vi "FRC Color Processing Example.vi"() -> ()   [LabVIEW 2025]
uses:
  <vilib>/Rock Robotics/WPI/Camera/WPI_CameraSettings Read MJPG.ctl
  <vilib>/Rock Robotics/WPI/Camera/WPI_CameraImageSize.ctl
  Vision Support Code/Camera Types.ctl
  <vilib>/Rock Robotics/WPI/Camera/WPI_CameraExposure Values.ctl
  <vilib>/Rock Robotics/WPI/Camera/WPI_CameraWhite Balance Values.ctl
  <vilib>/vision/NI_Vision_Development_Module.lvlib
panel:
  in  "Line Border":cluster{"Top":dbl, "Bottom":dbl}={"Top"=6.0, "Bottom"=1.0}
  in  "Use Calibration":bool=TRUE
  out "Instructions:":string="Use Source to load image files from a directory, or use a USB or IP camera connected to your laptop. Use Camera Settings 1 and 2 to achieve a dark image with bright and colorful stripes.\nLED Color can encoded as HSL or related color modes. Calibrate to the same color as the strips being reflected to the camera.\nClick and draw a line in Original Image to auto-calibrate the LED Color. You may want to widen and tweak Sat and Val by hand.\nThe Annotate button affects drawing a rectangle around the stripes and labeling it with a distance in ft. Distance relies on knowing the Camera Type and lens calibration (it looks up the lens view angle).\n\nAdjust Score Cutoff to make the code more or less picky. If the color is not very unique, you may need to increase the number of particles considered. The diagram uses a Size Limit to ignore colored things that are too small. You may need to adjust it if you are targetting from far away.\n\nResults give you the distance to the target, the center and box in a normalized (-1 to 1) and pixel coordinates.\n\nBe sure to read about setting camera exposure and brightness to help simplify your image and acquire color saturated images.\n\nThere are lots of comments on the diagram to explain the code."
  in  "Color Mode":u16(ring)=3 items=["RGB", "HSL", "HSV", "HSI"]
  in  "Particles":dbl=5.0
  in  "Score Cutoff %":dbl=70.0
  in  "Std Devs for Calibration":cluster{"H":dbl, "S":dbl, "V":dbl}={"H"=4.0, "S"=6.0, "V"=6.0}
  in  "Camera Type":T1=enum."MS HD3000 square"
  in  "image files":string[](array[string])
  out "Results":T2 {"Score" format="%#_3g"; "Pixels"."Rectangle"."Numeric 5" format="%#_3g"; "Pixels"."Rectangle"."Numeric 3" format="%#_3g"; "Pixels"."Rectangle"."Numeric 2" format="%#_3g"; "Pixels"."Rectangle"."Numeric" format="%#_3g"; "Normalized"."Rectangle"."Numeric 5" format="%#_2g"; "Normalized"."Rectangle"."Numeric 3" format="%#_2g"; "Normalized"."Rectangle"."Numeric 2" format="%#_2g"; "Normalized"."Rectangle"."Numeric" format="%#_2g"; "Normalized"."Center"."?" format="%#_3g"; "Normalized"."Center"."?" format="%#_3g"; "Distance (ft)" format="%#_3g"}
  in  "Source":enum32{"Files", "Camera"}(tab)
  in  "Images":i32(listbox)
  in  "Folder Location":path=path "C:/Program Files (x86)/National Instruments/LabVIEW 2016/examples/FRC/roboRIO/Vision/2017 Vision Example/Sample Images/LED Boiler"
  in  "Camera Settings":T3={"fps"=20, "compression"=30, "Image Size"=enum."320x240", "Config Shown"=FALSE}
  in  "Camera Address":string="USB 1"
  in  "Camera Settings 2":T7={"Exposure"=enum."Auto", "Exposure (%)"=50.0, "Brightness"=50, "White Balance"=enum."Auto", "Color Temp (K)"=0.0} {"Brightness" min=0 max=100}
  in  "Annotate":bool=TRUE
  out "Qualified Particles":i32
  in  "LED Color":T8={"Hue"={107.81818389892578, 139.81818389892578}, "Sat"={176.07142857142858, 255.0}, "Val"={40.53571428571429, 255.0}} {"Hue" scale=0.0..255.0 scale format="%#_3g"}
  out "Mask":T9(plugin-control)
  out "Original Image":T9(plugin-control)
  # "Legend:\n    Rectangle\n       Green - Good target, distance ft\n       Red - Bad target\n    Orange Text - Score in %"
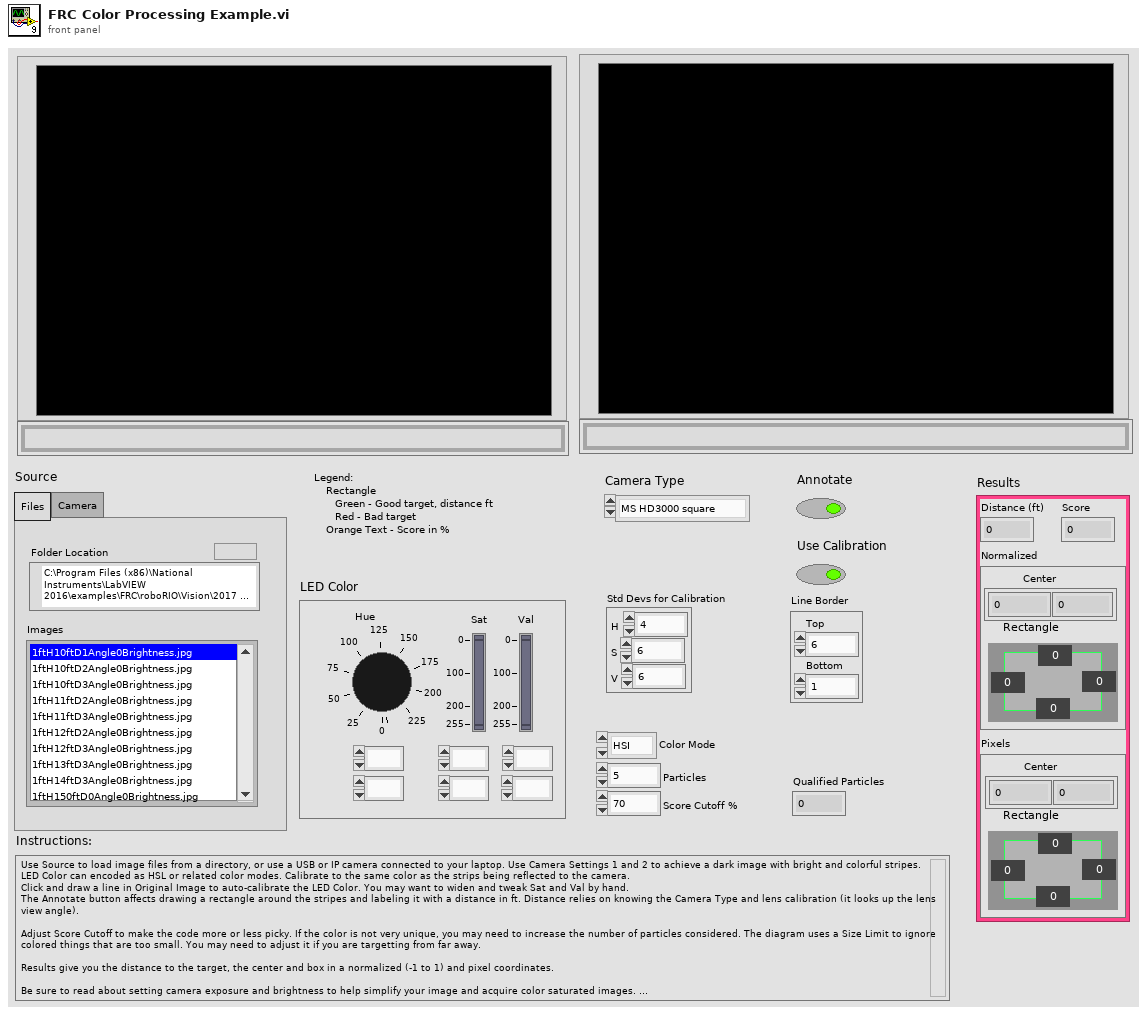
[diagram p1: front panel]
types:
  T1 = typedef "Camera Types.ctl" = enum16{"206", "1011", "1013", "MS HD3000 square", "MS HD3000 640x480"}
  T2 = cluster{"Distance (ft)":dbl, "Score":dbl, "Normalized":cluster{"Center":cluster{dbl, dbl}, "Rectangle":cluster{"Numeric":dbl, "Numeric 2":dbl, "Numeric 3":dbl, "Numeric 5":dbl}}, "Pixels":cluster{"Center":cluster{dbl, dbl}, "Rectangle":cluster{"Numeric":dbl, "Numeric 2":dbl, "Numeric 3":dbl, "Numeric 5":dbl}}}
  T3 = typedef "WPI_CameraSettings Read MJPG.ctl" = cluster{"fps":i32, "compression":i32, "Image Size":T4, "Config Shown":bool}
  T4 = typedef "WPI_CameraImageSize.ctl" = enum16{"640x480", "320x240", "160x120", "Custom"}
  T5 = typedef "WPI_CameraExposure Values.ctl" = enum16{"Auto", "Flicker-free 50 Hz", "Flicker-free 60 Hz", "Hold current", "Custom"}
  T6 = typedef "WPI_CameraWhite Balance Values.ctl" = enum16{"Auto", "Fixed indoor", "Fixed outdoor 1", "Fixed outdoor 2", "Fixed fluorescent 1", "Fixed fluorescent 2", "Hold current", "Custom"}
  T7 = cluster{"Exposure":T5, "Exposure (%)":dbl, "Brightness":i32, "White Balance":T6, "Color Temp (K)":dbl}
  T8 = cluster{"Hue":cluster{dbl, dbl}, "Sat":cluster{dbl, dbl}, "Val":cluster{dbl, dbl}}
  T9 = typedef "IMAQ Image.ctl" = refnum<image>
  T10 = typedef "Image Type" = u32
  T11 = typedef "Particle Parameters" = i32
  T12 = cluster{cluster{dbl, dbl}, cluster{dbl, dbl}, cluster{dbl, dbl}}
  T13 = cluster{"Left":dbl, "Top":dbl, "Right":dbl, "Bottom":dbl}
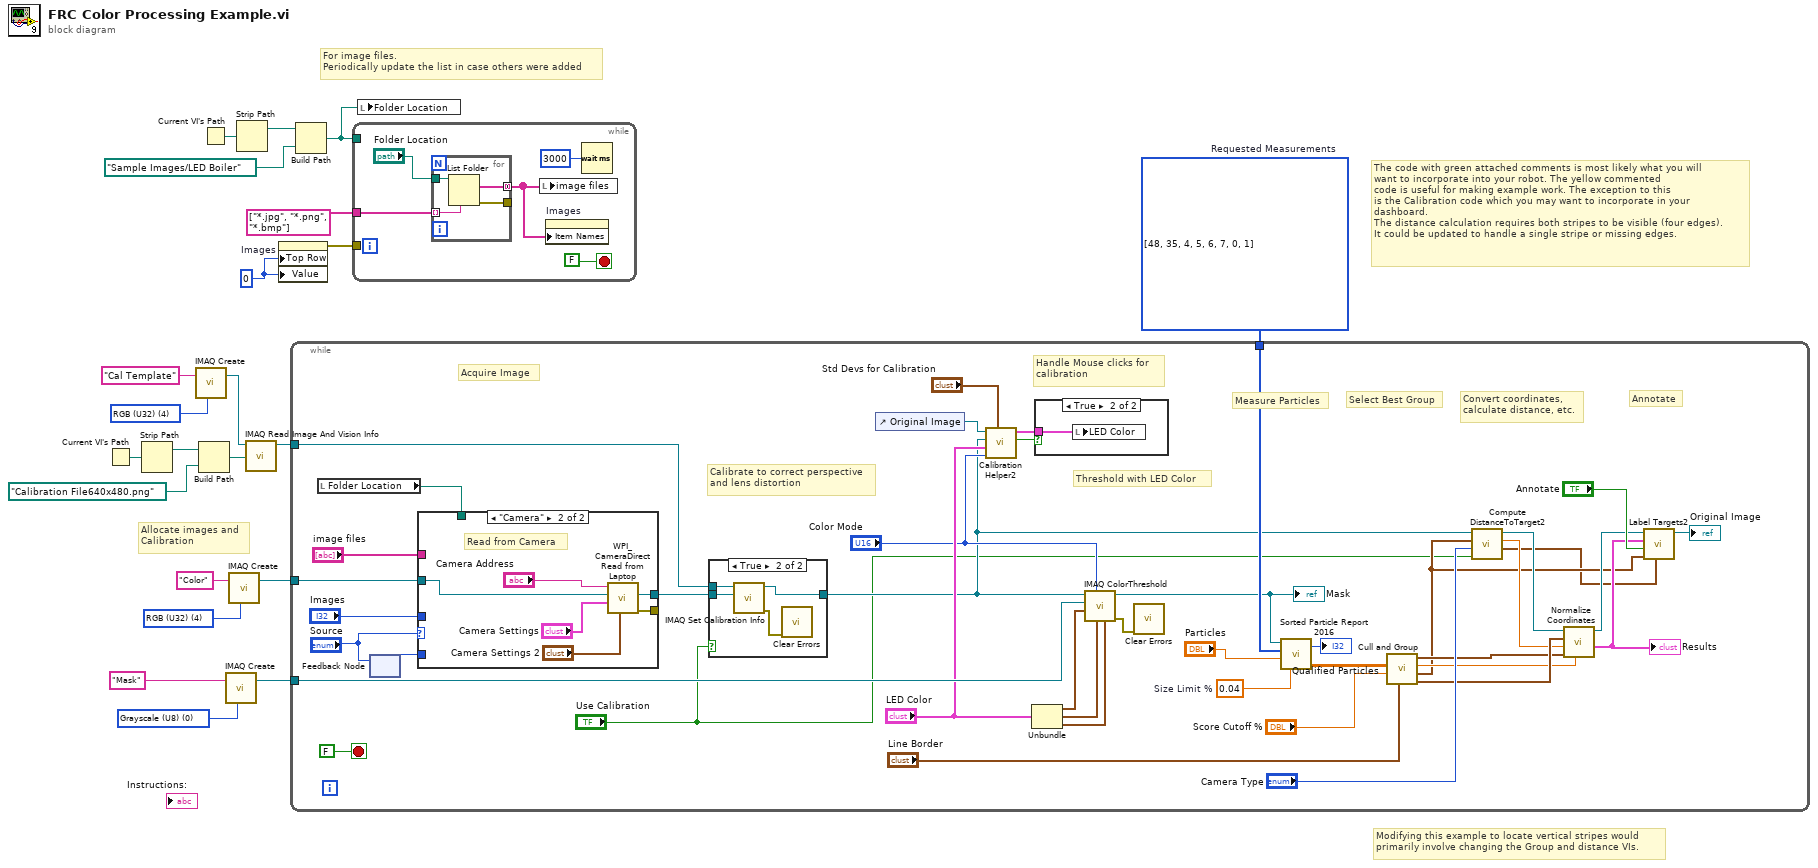
[diagram p0: block diagram]
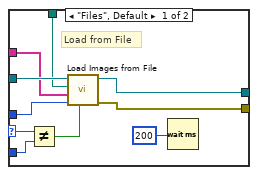
[diagram p4: hidden frame]
diagram:
  w8 = T10 4 items=["Grayscale (U8)", "Grayscale (I16)", "Grayscale (SGL)", "Complex (CSG)", "RGB (U32)", "HSL (U32)", "RGB (U64)", "Grayscale (U16)"] ("Image Type")
  w11 = u32 0 ("milliseconds to wait")
  w17 = T11[] [48, 35, 4, 5, 6, 7, 0, 1] items=["Center of Mass X", "Center of Mass Y", "First Pixel X", "First Pixel Y", "Bounding Rect Left", "Bounding Rect Top", "Bounding Rect Right", "Bounding Rect Bottom", "Max Feret Diameter Start X", "Max Feret Diameter Start Y", "Max Feret Diameter End X", "Max Feret Diameter End Y", "Max Horiz. Segment Length Left", "Max Horiz. Segment Length Right", "Max Horiz. Segment Length Row", "-", "Bounding Rect Width", "Bounding Rect Height", "Bounding Rect Diagonal", "Perimeter", "Convex Hull Perimeter", "Holes' Perimeter", "Max Feret Diameter", "Equivalent Ellipse Major Axis", "Equivalent Ellipse Minor Axis", "Equivalent Ellipse Minor Axis (Feret)", "Equivalent Rect Long Side", "Equivalent Rect Short Side", "Equivalent Rect Diagonal", "Equivalent Rect Short Side (Feret)", "Average Horiz. Segment Length", "Average Vert. Segment Length", "Hydraulic Radius", "Waddel Disk Diameter", "-", "Area", "Holes' Area", "Particle & Holes' Area", "Convex Hull Area", "Image Area", "-", "Number of Holes", "Number of Horiz. Segments", "Number of Vert. Segments", "-", "Orientation", "Max Feret Diameter Orientation", "-", "% Area/Image Area", "% Area/(Particle & Holes' Area)", "Ratio of Equivalent Ellipse Axes", "Ratio of Equivalent Rect Sides", "-", "Elongation Factor", "Compactness Factor", "Heywood Circularity Factor", "Type Factor", "-", "Sum X", "Sum Y", "Sum XX", "Sum XY", "Sum YY", "Sum XXX", "Sum XXY", "Sum XYY", "Sum YYY", "-", "Moment of Inertia XX", "Moment of Inertia XY", "Moment of Inertia YY", "Moment of Inertia XXX", "Moment of Inertia XXY", "Moment of Inertia XYY", "Moment of Inertia YYY", "Norm. Moment of Inertia XX", "Norm. Moment of Inertia XY", "Norm. Moment of Inertia YY", "Norm. Moment of Inertia XXX", "Norm. Moment of Inertia XXY", "Norm. Moment of Inertia XYY", "Norm. Moment of Inertia YYY", "Hu Moment 1", "Hu Moment 2", "Hu Moment 3", "Hu Moment 4", "Hu Moment 5", "Hu Moment 6", "Hu Moment 7"]  # Requested Measurements
  w20 = T10 0 items=["Grayscale (U8)", "Grayscale (I16)", "Grayscale (SGL)", "Complex (CSG)", "RGB (U32)", "HSL (U32)", "RGB (U64)", "Grayscale (U16)"] ("Image Type")
  w21 = T10 4 items=["Grayscale (U8)", "Grayscale (I16)", "Grayscale (SGL)", "Complex (CSG)", "RGB (U32)", "HSL (U32)", "RGB (U64)", "Grayscale (U16)"] ("Image Type")
  # "Modifying this example to locate vertical stripes would\nprimarily involve changing the Group and distance VIs."
  # "The code with green attached comments is most likely what you will\nwant to incorporate into your robot. The yellow commented\ncode is useful for making example work. The exception to this\nis the Calibration code which you may want to incorporate in your\ndashboard.\nThe distance calculation requires both stripes to be visible (four edges).\nIt could be updated to handle a single stripe or missing edges."
  # "For image files.\nPeriodically update the list in case others were added"
  # "Allocate images and\nCalibration"
  n1 = Current VI's Path() -> (path=w4:path)
  n2 = Strip Path(path=w4) -> (stripped path=w1:path)  [unwired: 1 out]
  n3 = call "IMAQ Create"("Image Name"="Cal Template", "Image Type"=w8) -> ("New Image"=w6:T9)  [unwired: 2 in, 2 out]
  n4 = Build Path(base path=w1, name or relative path=path "Calibration File640x480.png" ("Folder Location")) -> (appended path=w3:path)
  n5 = Current VI's Path() -> (path=w16:path)
  n6 = call "IMAQ Create"("Image Name"="Mask", "Image Type"=w20) -> ("New Image"=w18:T9)  [unwired: 2 in, 2 out]
  n7 = call "IMAQ Create"("Image Name"="Color", "Image Type"=w21) -> ("New Image"=w9:T9)  [unwired: 2 in, 2 out]
  n8 = Strip Path(path=w16) -> (stripped path=w14:path)  [unwired: 1 out]
  n9 = call "IMAQ Read Image And Vision Info"("File Path"=w3, "Image"=w6) -> ("Image Out"=w5:T9)  [unwired: 7 in, 2 out]
  n10 = property on="Images" class="LstBox (strict)"("Top Row"=w11, "Value"=w11) -> (error out=w12:errorcluster)  [unwired: 2 in, 1 out]
  n11 = while {
    tunnel: w9 -> [w63]
    tunnel: w18 -> [w61]
    tunnel: w17 -> [w57]
    tunnel: w5 -> [w25]
    stop <- FALSE stop-if-true
    w55 = 0.04  # Size Limit %
    # "Calibrate to correct perspective\nand lens distortion"
    # "Handle Mouse clicks for\ncalibration"
    # "Measure Particles"
    # "Convert coordinates,\ncalculate distance, etc."
    # "Annotate"
    # "Select Best Group"
    # "Threshold with LED Color"
    # "Acquire Image"
    n12 = local read "Folder Location"() -> (w45:path)
    n13 = feedback-in #1("Source") -> ()
    n14 = feedback #1() -> (w43:enum32{"Files", "Camera"})  [unwired: 1 in]
    n15 = case shown="\"Camera\"" "Source" {
      selector: "Source" -> [w73 _]
      tunnel: [w79 w86] -> _
      tunnel: [w80 w85] -> w26
      tunnel: w63 -> [w78 w84]
      tunnel: "image files" -> [w75 _]
      tunnel: "Images" -> [w77 _]
      tunnel: w45 -> [w76 _]
      tunnel: w43 -> [w72 _]
      frame "Files", Default {
        # "Load from File"
        n16 = Not Equal?(x=w73, y=w72) -> (x != y?=w71:bool)
        n17 = call "Load Images from File.vi"("Force Load"=w71, "Images"=w77, "image files"=w75, "Folder Location"=w76, "Refnum in"=w78) -> ("error out"=w79:errorcluster, "Refnum out"=w80:T9)  [unwired: 5 in]
        n18 = Wait (ms)(milliseconds to wait=u32 200 ("delay (ms)")) -> ()  [unwired: 1 out]
      }
      frame "Camera" {
        # "Read from Camera"
        n19 = call <vilib>:"WPI_CameraDirect Read from Laptop.vi"("Camera Settings 2"="Camera Settings 2", "Camera Settings"="Camera Settings", "Image"=w84, "address"="Camera Address") -> ("error out"=w86:errorcluster, "Image Out"=w85:T9)  [unwired: 6 in]
      }
    }
    n20 = case shown="True" "Use Calibration" {
      tunnel: [w65 w69] -> w27
      tunnel: w26 -> [w65 w68]
      tunnel: w25 -> [_ w67]
      frame False {
      }
      frame True {
        n21 = call "IMAQ Set Calibration Info"("Image Dst"=w68, "Image Src"=w67) -> ("error out"=w66:errorcluster, "Calibrated Image"=w69:T9)  [unwired: 8 in]
        n22 = call <vilib>:"Clear Errors.vi"("error in (no error)"=w66) -> ()  [unwired: 5 in, 2 out]
      }
    }
    n23 = control-ref of="Original Image"() -> (w50:refnum<vi>)
    n24 = call "Calibration Helper2.vi"("Std Devs"="Std Devs for Calibration", "Color Mode"="Color Mode", "Color Components"="LED Color", "Image"=w27, "Image Ctl Refnum"=w50) -> ("Changed"=w49:bool, "output color"=w48:T12)  [unwired: 5 in]
    n25 = Unbundle("LED Color") -> ("Hue"=w60:cluster{dbl, dbl}, "Sat"=w59:cluster{dbl, dbl}, "Val"=w58:cluster{dbl, dbl})
    n26 = case shown="True" w49 {
      tunnel: w48 -> [_ w70]
      frame False {
      }
      frame True {
        n27 = local write "LED Color"(w70) -> ()
      }
    }
    n28 = call "IMAQ ColorThreshold"("Blue or Luma or Val or Inten Range"=w58, "Green or Sat Range"=w59, "Color Mode"="Color Mode", "Red or Hue Range"=w60, "Image Dst"=w61, "Image Src"=w27) -> ("error out"=w51:errorcluster, "Image Dst Out"=w40:T9)  [unwired: 4 in]
    "Mask" <- w40
    n29 = call <vilib>:"Clear Errors.vi"("error in (no error)"=w51) -> ()  [unwired: 5 in, 2 out]
    n30 = call "Sorted Particle Report 2016.vi"("Min Area Size %"=w55, "Particle Count Limit"="Particles", "Pixel Measurements"=w57, "Image in"=w40) -> ("Sorted Data"=w42:dbl[][], "Particles"=→"Qualified Particles":i32)
    n31 = call "Cull and Group.vi"("Line Border"="Line Border", "Score Cutoff"="Score Cutoff %", "Sorted Data"=w42) -> ("Rect"=w38:T13, "Line"=w29:T13, "Score"=w32:dbl, "Center"=w34:cluster{"X":dbl, "Y":dbl})  [unwired: 5 in]
    n32 = call "Compute DistanceToTarget2.vi"("Calibrated"="Use Calibration", "Camera Type"="Camera Type", "Line"=w29, "Image Src"=w27) -> ("Edges"=w28:cluster{"X":sgl, "Y":sgl}[], "Distance (ft)"=w37:dbl, "Image Dst Out"=w36:T9)  [unwired: 5 in]
    n33 = call "Normalize Coordinates.vi"("Score"=w32, "Center"=w34, "Distance"=w37, "Bounding box"=w38, "Image in"=w36) -> ("Results"=w33:T2, "Image out"=w35:T9)  [unwired: 5 in]
    "Results" <- w33
    n34 = call "Label Targets2.vi"("Edges"=w28, "Line"=w29, "Annotate"="Annotate", "Results"=w33, "Image in"=w35) -> ("Image out"=→"Original Image":T9)  [unwired: 6 in]
  }
  n35 = Build Path(base path=w14, name or relative path=path "Sample Images/LED Boiler" ("Folder Location")) -> (appended path=w13:path)
  n36 = while {
    tunnel: w13 -> [_]
    tunnel: w12 -> [_]
    tunnel: string[] ["*.jpg", "*.png", "*.bmp"] -> [w87]
    stop <- FALSE stop-if-true
    n37 = for {
      tunnel: [w95] -> w89 mode=concatenating
      tunnel: "Folder Location" -> [w94]
      tunnel: [w93] -> _
      tunnel: w87 -> [w92] mode=indexing
      n38 = List Folder(path=w94, pattern=w92) -> (filenames=w95:string[], error out=w93:errorcluster)  [unwired: 2 in, 2 out]
    }
    n39 = local write "image files"(w89) -> ()
    n40 = property on="Images" class="LstBox (strict)"("Item Names"=w89) -> ()  [unwired: 2 in, 2 out]
    n41 = Wait (ms)(milliseconds to wait=u32 3000) -> ()  [unwired: 1 out]
  }
  n42 = local write "Folder Location"(w13) -> ()
